vi "moving average.vi"(10 "average over x points":i32=3, 11 "Array":dbl[](array[numeric])) -> (2 "array index":i32[](array[numeric]), 3 "moving average array":dbl[](array[numeric]))   [LabVIEW 2019]
panel:
  out "XY Graph":cluster{i32[], dbl[]}[](graph)
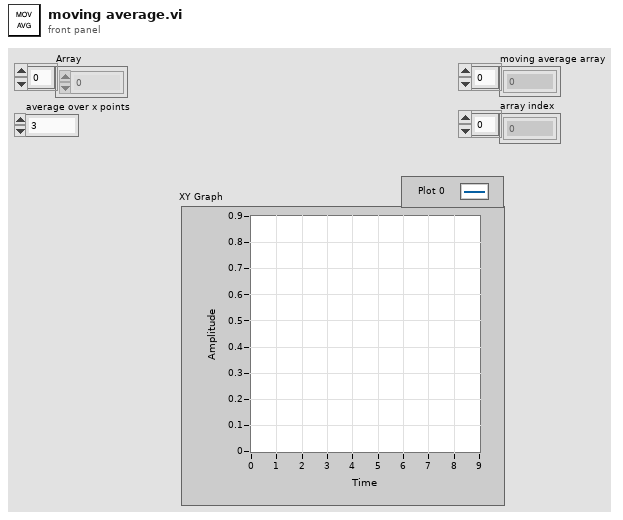
[diagram p1: front panel]
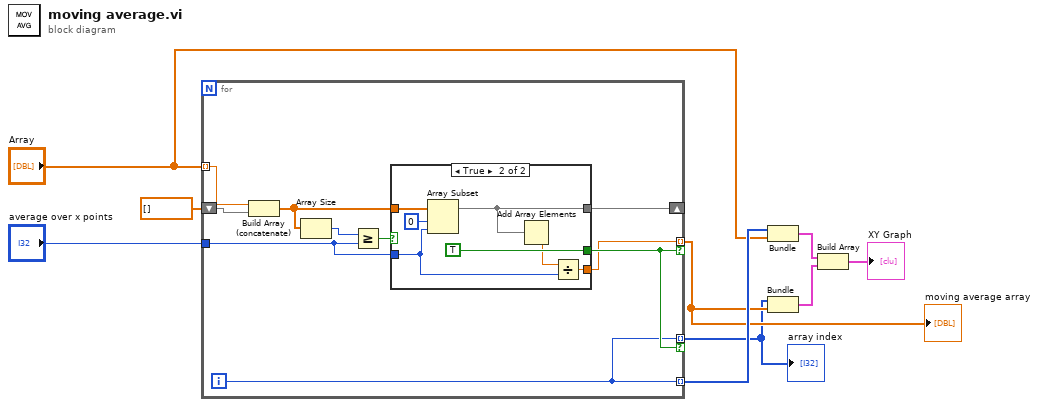
[diagram p0: block diagram]
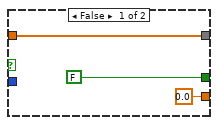
[diagram p2: hidden frame]
diagram:
  n1 = for {
    tunnel: "Array" -> [w19] mode=indexing
    shift-right: [w13] -> _
    shift-left: dbl[] [] -> [w18]
    tunnel: "average over x points" -> [w14]
    tunnel: [w11] -> w6 mode=indexing if=w12
    tunnel: [w10] -> w7 mode=indexing
    tunnel: [w10] -> w5 mode=indexing if=w12
    i -> [w10]
    n2 = Build Array (concatenate)(w19, w18) -> (w17:dbl[])
    n3 = Array Size(array=w17) -> (size(s)=w16:i32)
    n4 = Greater Or Equal?(x=w16, y=w14) -> (x >= y?=w15:bool)
    n5 = case shown="True" w15 {
      tunnel: [w22 w26] -> w13
      tunnel: w17 -> [w22 w29]
      tunnel: w14 -> [_ w24]
      tunnel: [FALSE TRUE] -> w12
      tunnel: [0.0 w23] -> w11
      frame False {
      }
      frame True {
        n6 = Array Subset(array=w29, index=0, length=w24) -> (w26:dbl[])
        n7 = Add Array Elements(numeric array=w26) -> (sum=w25:dbl)
        n8 = Divide(x=w25, y=w24) -> (x/y=w23:dbl)
      }
    }
  }
  "moving average array" <- w6
  "array index" <- w5
  n9 = Bundle(w7, "Array"="Array") -> (w4:cluster{i32[], "Array":dbl[]})  [unwired: 1 in]
  n10 = Bundle(w5, w6) -> (w3:cluster{i32[], dbl[]})  [unwired: 1 in]
  n11 = Build Array(w4, w3) -> (→"XY Graph":cluster{i32[], "Array":dbl[]}[])
